vi "uart data_main.vi"() -> ()   [LabVIEW 2015]
uses:
  data_typedef.ctl
  <vilib>/Instr/_visa.llb/VISA Configure Serial Port (Instr).vi
panel:
  out "Accelero Chart":T1(graph)
  out "Temperature Chart":dbl[](graph)
  in  "stop":bool
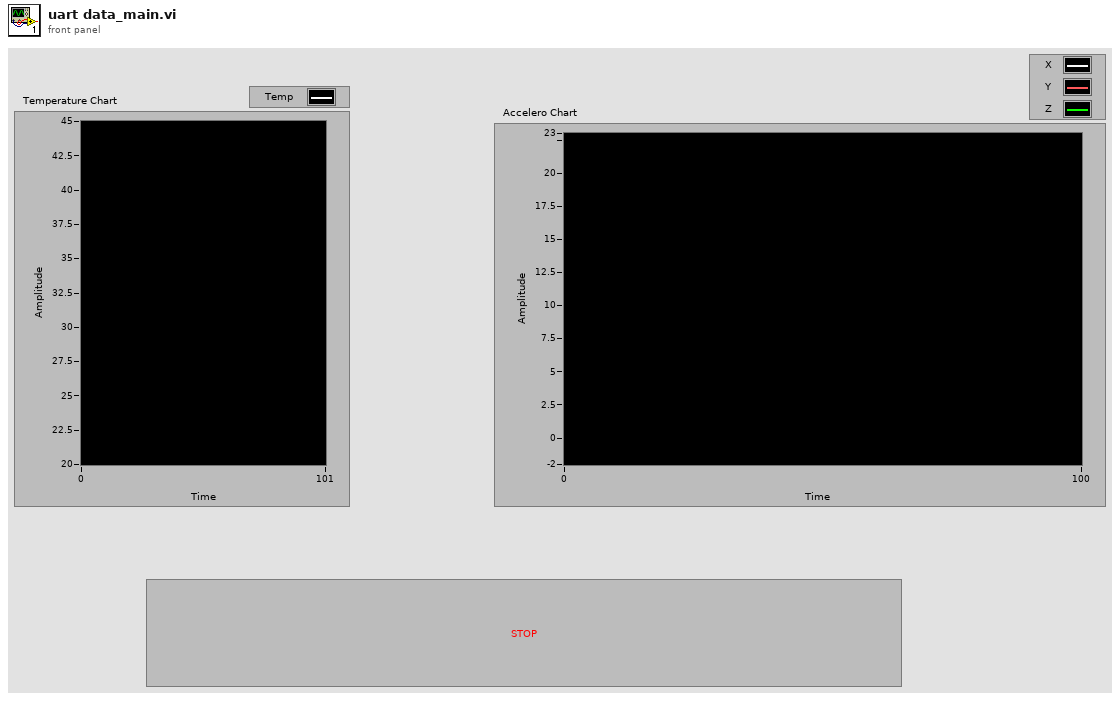
[diagram p1: front panel]
types:
  T1 = cluster{"X element out":dbl, "X element out":dbl, "Z element out":dbl}
  T2 = cluster{"Z element out":dbl, "X element out":dbl, "X element out 2":dbl}[]
  T3 = typedef "data_typedef.ctl" = cluster{"Accelero Array":dbl[], "Z out":dbl[], "Y out":dbl[], "X out":dbl[], "Numeric":i32}
  T4 = typedef "enum_typedef.ctl" = enum16{"Temperature", "X axis", "Y axis", "Z axis"}
  T5 = cluster{"X element out":dbl, "Y element out":dbl, "Z element out":dbl}
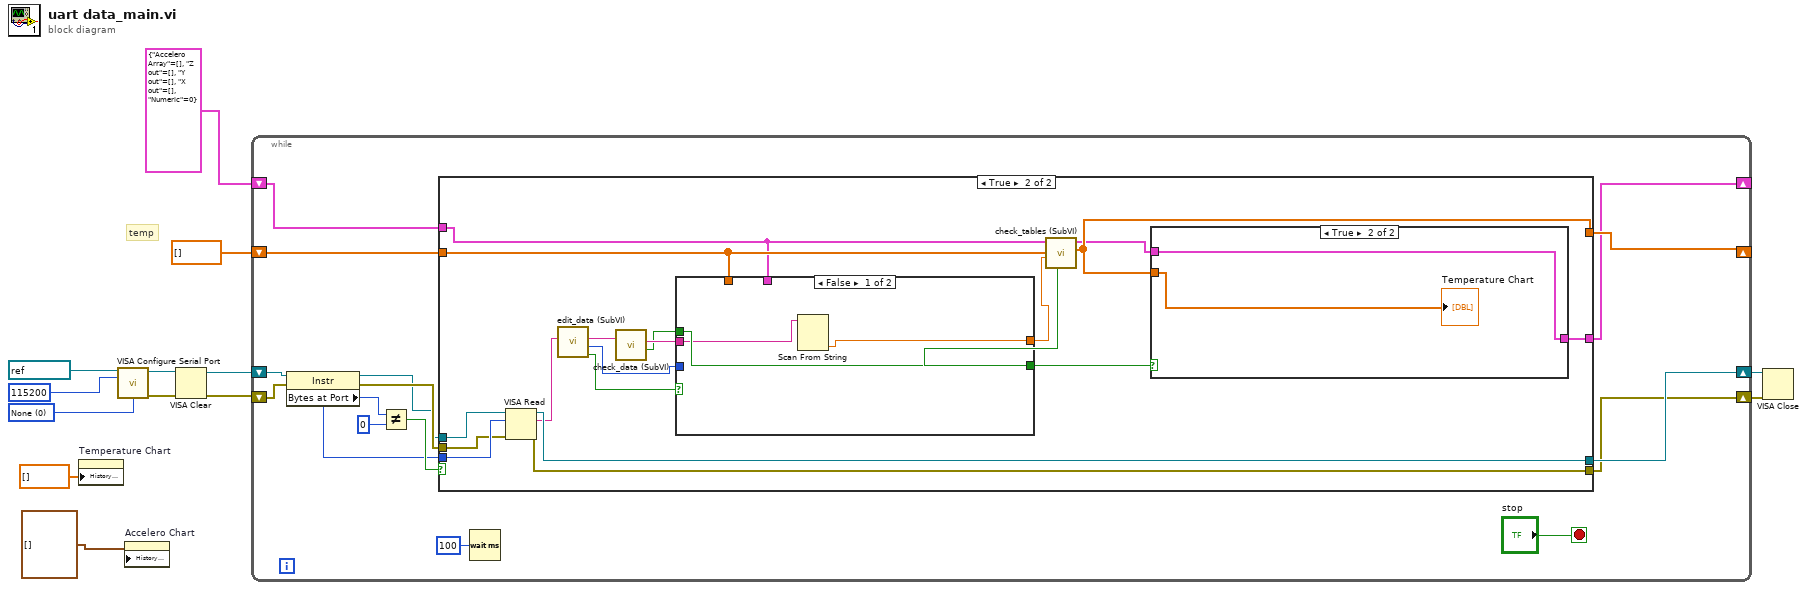
[diagram p0: block diagram]
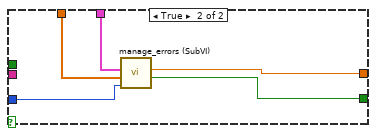
[diagram p3: hidden frame]
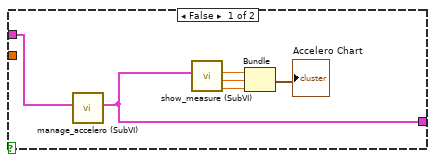
[diagram p4: hidden frame]
diagram:
  w9 = u16 0 items=["None", "XON/XOFF", "RTS/CTS", "XON/XOFF & RTS/CTS", "DTR/DSR", "XON/XOFF & DTR/DSR"] ("flow control (0:none)")
  # "temp"
  n1 = property on="Temperature Chart" class="WFChart (strict)"("History Data"=dbl[] []) -> ()  [unwired: 2 in, 2 out]
  n2 = call-poly "VISA Configure Serial Port"("VISA resource name"=refnum<visa-resource-name> "COM5", "baud rate (9600)"=u32 115200, "flow control (0:none)"=w9) -> ("VISA resource name out"=w5:refnum<visa-resource-name>, "error out"=w4:errorcluster)  [unwired: 11 in]
  n3 = property on="Accelero Chart" class="WFChart (strict)"("History Data"=T2 []) -> ()  [unwired: 2 in, 2 out]
  n4 = VISA Clear(VISA resource name=w5, error in (no error)=w4) -> (VISA resource name out=w6:refnum<visa-resource-name>, error out=w7:errorcluster)
  n5 = while {
    shift-right: [w27] -> w11
    shift-left: w6 -> [w26]
    shift-right: [w23] -> w10
    shift-left: w7 -> [w24]
    shift-right: [w16] -> _
    shift-left: dbl[] [] -> [w19]
    shift-right: [w14] -> _
    shift-left: T3 {"Accelero Array"=[], "Z out"=[], "Y out"=[], "X out"=[], "Numeric"=0} ("Tabs") -> [w15]
    stop <- "stop" stop-if-true
    # "main loop"
    n6 = property class="Instr"(reference=w26, error in=w24) -> (reference out=w22:refnum<visa-resource-name>, error out=w25:errorcluster, "Bytes at Port"=w18:u32)
    n7 = Not Equal?(x=w18, y=u32 0) -> (x != y?=w20:bool)
    n8 = case shown="True" w20 {
      tunnel: [w32 w50] -> w27
      tunnel: w18 -> [_ w49]
      tunnel: w25 -> [w31 w48]
      tunnel: [w31 w47] -> w23
      tunnel: w22 -> [w32 w46]
      tunnel: w19 -> [w30 w39]
      tunnel: [w30 w44] -> w16
      tunnel: w15 -> [w29 w36]
      tunnel: [w29 w43] -> w14
      frame False {
      }
      frame True {
        # "true"
        n9 = VISA Read(VISA resource name=w46, byte count=w49, error in (no error)=w48) -> (VISA resource name out=w50:refnum<visa-resource-name>, read buffer=w33:string, error out=w47:errorcluster)  [unwired: 1 out]
        n10 = call "edit_data (SubVI).vi"("data in"=w33) -> ("error bool out"=w34:bool, "Enum"=w35:T4, "data out"=w45:string)  [unwired: 8 in]
        n11 = call "check_data (SubVI).vi"("read buffer"=w45) -> ("buffer out"=w41:string, "bool out"=w40:bool)  [unwired: 8 in]
        n12 = case shown="False" w34 {
          tunnel: w41 -> [w52 _]
          tunnel: w40 -> [w53 _]
          tunnel: w39 -> [_ w57]
          tunnel: [w53 w58] -> w38
          tunnel: [w51 w54] -> w37
          tunnel: w35 -> [_ w56]
          tunnel: w36 -> [_ w55]
          frame False {
            n13 = Scan From String(input string=w52) -> (output 1=w51:dbl)  [unwired: 4 in, 3 out]
          }
          frame True {
            n14 = call "manage_errors (SubVI).vi"("Enum"=w56, "Temperature Array"=w57, "Data in"=w55) -> ("Boolean out"=w58:bool, "Out value"=w54:dbl)  [unwired: 7 in]
          }
        }
        n15 = call "check_tables (SubVI).vi"("bool in"=w38, "numeric buffer in"=w37, "temperature array in"=w39, "Data in"=w36) -> ("temperature array out"=w44:dbl[], "Data out"=w42:T3)  [unwired: 6 in]
        n16 = case shown="True" w38 {
          tunnel: w44 -> [_ w66]
          tunnel: w42 -> [w60 w65]
          tunnel: [w59 w65] -> w43
          frame False {
            n17 = call "manage_accelero (SubVI).vi"("Data in"=w60) -> ("Data out"=w59:T3)  [unwired: 9 in]
            n18 = call "show_measure (SubVI).vi"("Data in"=w59) -> ("Z element out"=w63:dbl, "Y element out"=w61:dbl, "X element out"=w64:dbl)  [unwired: 8 in]
            n19 = Bundle("X element out"=w64, "Y element out"=w61, "Z element out"=w63) -> (→"Accelero Chart":T5)  [unwired: 1 in]
          }
          frame True {
            "Temperature Chart" <- w66
          }
        }
      }
    }
    n20 = Wait (ms)(milliseconds to wait=u32 100) -> ()  [unwired: 1 out]
  }
  n21 = VISA Close(VISA resource name=w11, error in (no error)=w10) -> ()  [unwired: 1 out]
